vi "Gün sayacı.vi"() -> ()   [LabVIEW 2014]
panel:
  out "GÜN":string
  in  "SAYI":dbl
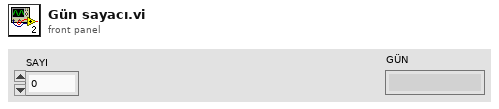
[diagram p1: front panel]
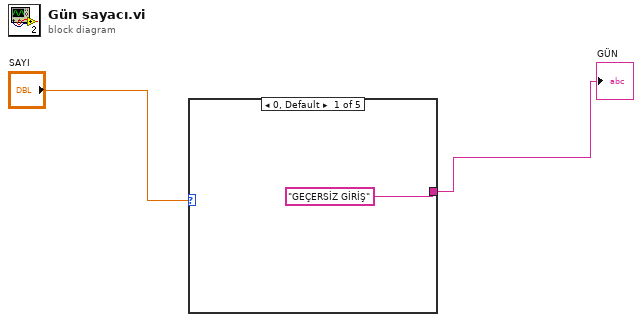
[diagram p0: block diagram]
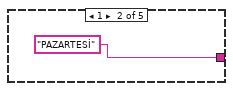
[diagram p2: hidden frame]
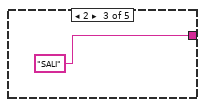
[diagram p3: hidden frame]
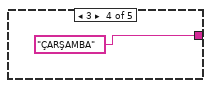
[diagram p4: hidden frame]
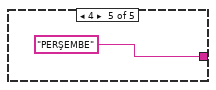
[diagram p5: hidden frame]
diagram:
  n1 = case shown="0, Default" "SAYI" {
    tunnel: ["GEÇERSİZ GİRİŞ" "PAZARTESİ" "SALI" "ÇARŞAMBA" "PERŞEMBE"] -> w1
    frame 0, Default {
    }
    frame 1 {
    }
    frame 2 {
    }
    frame 3 {
    }
    frame 4 {
    }
  }
  "GÜN" <- w1
